vi "Rpt _Get _Repair Data.vi"(0 "Traceability 引用句柄":refnum<k24>, 1 "Model":string, 2 "DateFrom":string, 3 "DateTo":string, 4 "DateCode":string, 5 "ItemNo":string, 6 "CompanyCode":string, 7 "error in (no error)":errorcluster caption="错误输入（无错误）", 8 "CauseCode":string, 9 "TestStation":string, 10 "ProductType":string, 11 "Location":string, 12 "UserNo":string, 13 "IntSerialNo":string) -> (20 "Traceability 引用句柄输出":refnum<k24>, 21 ".NET:System.Data.DataSet":T1={"CaseSensitive"=FALSE, "Container"=refnum, "DataSetName"="", "DefaultViewManager"=refnum, "DesignMode"=FALSE, "EnforceConstraints"=FALSE, "ExtendedProperties"=refnum, "HasErrors"=FALSE, "IsInitialized"=FALSE, "Locale"=refnum, "Namespace"="", "Prefix"="", "Relations"=refnum, "RemotingFormat"=0, "SchemaSerializationMode"=1, "Site"=refnum, "Tables"=refnum} {"SchemaSerializationMode" items=["IncludeSchema"=1, "ExcludeSchema"=2]; "RemotingFormat" items=["Xml", "Binary"]}, 27 "error out":errorcluster caption="错误输出")   [LabVIEW 2014, in "Traceability.lvlib"]
uses:
  D:/webservice/Traceability.dll
  Traceability.dll
  System.Data
  Traceability.lvlib
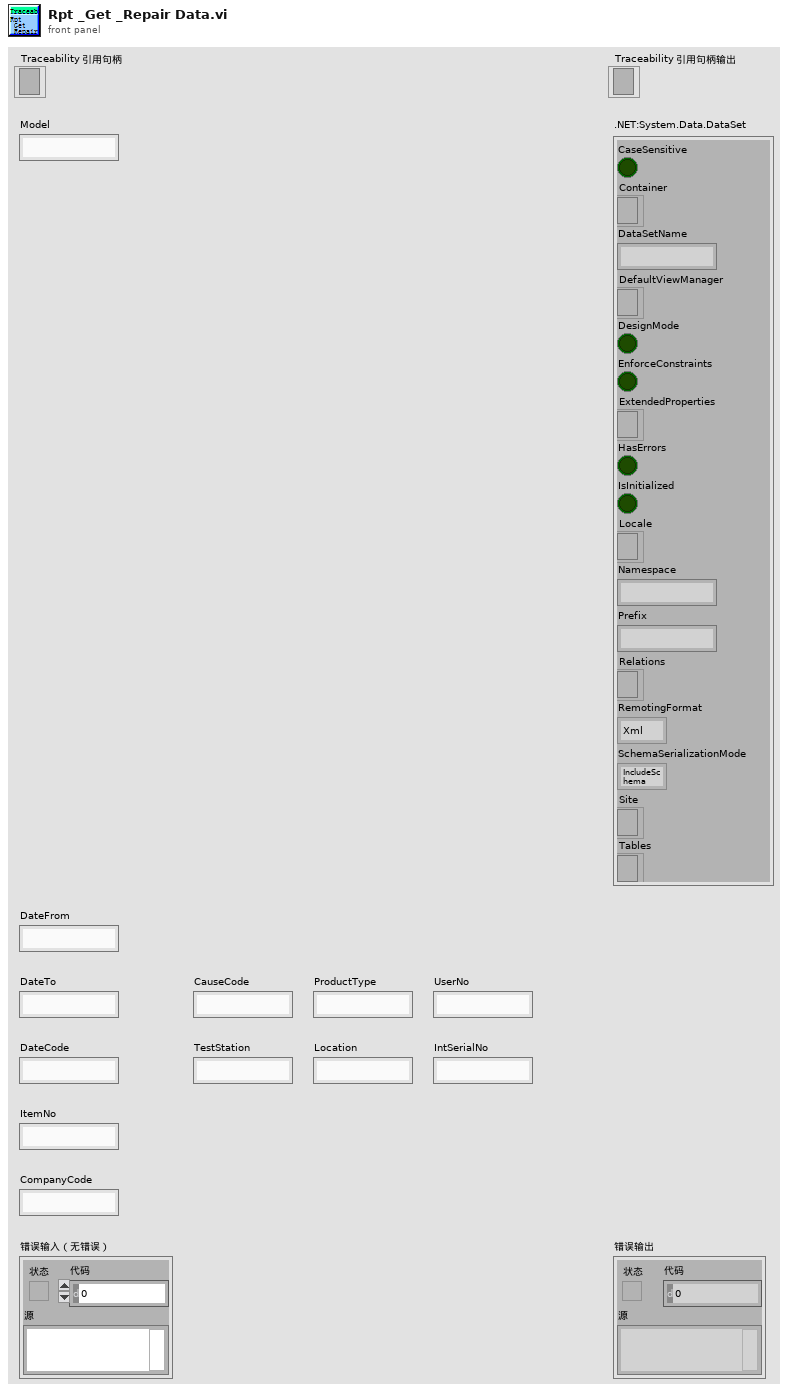
[diagram p1: front panel]
types:
  T1 = cluster{"CaseSensitive":bool, "Container":refnum<k24>, "DataSetName":string, "DefaultViewManager":refnum<k24>, "DesignMode":bool, "EnforceConstraints":bool, "ExtendedProperties":refnum<k24>, "HasErrors":bool, "IsInitialized":bool, "Locale":refnum<k24>, "Namespace":string, "Prefix":string, "Relations":refnum<k24>, "RemotingFormat":i32, "SchemaSerializationMode":i32, "Site":refnum<k24>, "Tables":refnum<k24>}
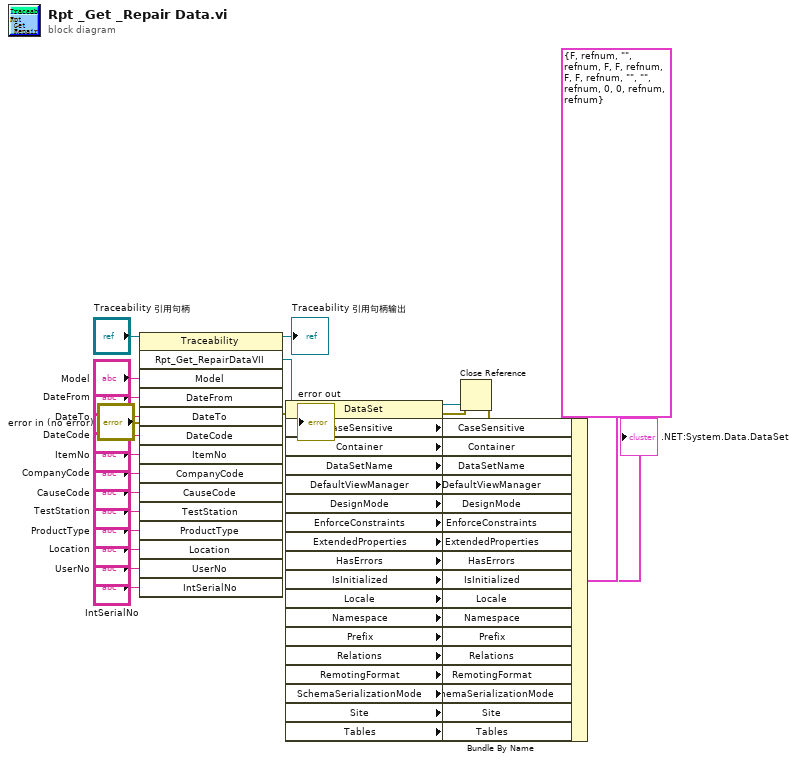
[diagram p0: block diagram]
diagram:
  n1 = invoke class="Traceability" method="Rpt_Get_RepairDataVII"(reference="Traceability 引用句柄", error in="error in (no error)", "Model"="Model", "DateFrom"="DateFrom", "DateTo"="DateTo", "DateCode"="DateCode", "ItemNo"="ItemNo", "CompanyCode"="CompanyCode", "CauseCode"="CauseCode", "TestStation"="TestStation", "ProductType"="ProductType", "Location"="Location", "UserNo"="UserNo", "IntSerialNo"="IntSerialNo") -> (reference out=→"Traceability 引用句柄输出":refnum<k24>, error out=w4:errorcluster, "Rpt_Get_RepairDataVII"=w36:refnum<k24>)  [unwired: 1 in, 12 out]
  n2 = property class="DataSet"(reference=w36, error in=w4) -> (reference out=w3:refnum<k24>, error out=w2:errorcluster, "CaseSensitive"=w33:bool, "Container"=w32:refnum<k24>, "DataSetName"=w31:string, "DefaultViewManager"=w30:refnum<k24>, "DesignMode"=w29:bool, "EnforceConstraints"=w28:bool, "ExtendedProperties"=w27:refnum<k24>, "HasErrors"=w26:bool, "IsInitialized"=w25:bool, "Locale"=w24:refnum<k24>, "Namespace"=w23:string, "Prefix"=w22:string, "Relations"=w21:refnum<k24>, "RemotingFormat"=w20:i32, "SchemaSerializationMode"=w19:i32, "Site"=w18:refnum<k24>, "Tables"=w17:refnum<k24>)
  n3 = Bundle By Name(cluster=T1 {"CaseSensitive"=FALSE, "Container"=refnum, "DataSetName"="", "DefaultViewManager"=refnum, "DesignMode"=FALSE, "EnforceConstraints"=FALSE, "ExtendedProperties"=refnum, "HasErrors"=FALSE, "IsInitialized"=FALSE, "Locale"=refnum, "Namespace"="", "Prefix"="", "Relations"=refnum, "RemotingFormat"=0, "SchemaSerializationMode"=0, "Site"=refnum, "Tables"=refnum} (".NET:System.Data.DataSet"), "CaseSensitive"=w33, "Container"=w32, "DataSetName"=w31, "DefaultViewManager"=w30, "DesignMode"=w29, "EnforceConstraints"=w28, "ExtendedProperties"=w27, "HasErrors"=w26, "IsInitialized"=w25, "Locale"=w24, "Namespace"=w23, "Prefix"=w22, "Relations"=w21, "RemotingFormat"=w20, "SchemaSerializationMode"=w19, "Site"=w18, "Tables"=w17) -> (→".NET:System.Data.DataSet":T1)
  n4 = Close Reference(reference=w3, error in (no error)=w2) -> (error out=→"error out":errorcluster)
